vi "Set Default Characteristics.vi"(8 "error in (no error)":errorcluster, 11 "5105 in":refnum<class "5105.lvclass">) -> (0 "error out":errorcluster, 3 "5105 out":refnum<class "5105.lvclass">)   [LabVIEW 2019, in "5105.lvlib" / "5105.lvclass"]
uses:
  5105.lvclass
  C:/Users/rdexter/Documents/Development/PPL/Oscilloscope.lvlibp/Oscilloscope.lvclass
  builds/Instruments/Oscilloscope.lvlibp/Custom Controls/Trigger Modifier.ctl
  builds/Instruments/Oscilloscope.lvlibp/Custom Controls/Trigger Type.ctl
  builds/Instruments/Oscilloscope.lvlibp/Accessors/Read Trigger Settings.vi
  builds/Instruments/Oscilloscope.lvlibp/Accessors/Read Horizontal Setting.vi
  builds/Instruments/Oscilloscope.lvlibp/Accessors/Read Channel Setting.vi
  builds/Instruments/Oscilloscope.lvlibp/Accessors/Write Trigger Settings.vi
  builds/Instruments/Oscilloscope.lvlibp/Accessors/Write Horizontal Setting.vi
  builds/Instruments/Oscilloscope.lvlibp/Accessors/Write Channel Settings.vi
  builds/Instruments/Oscilloscope.lvlibp/Oscilloscope.lvclass
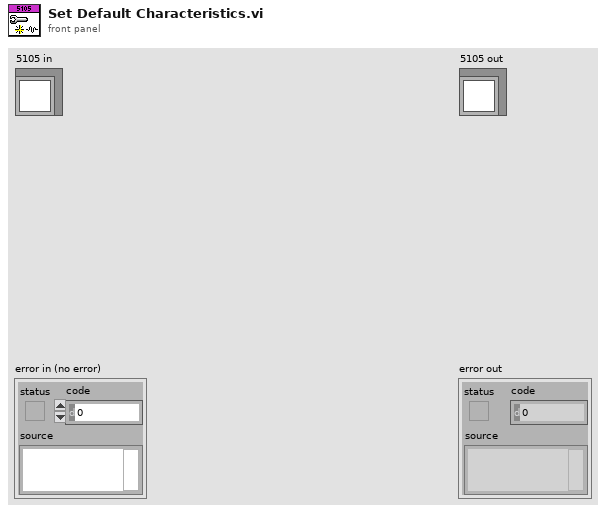
[diagram p1: front panel]
types:
  T1 = typedef "Oscilloscope.lvlibp/Oscilloscope.lvclass/Trigger Type.ctl" = enum16{"Immediate", "Analog Edge", "Digital", "Window", "Hysteresis"}
  T2 = typedef "Oscilloscope.lvlibp/Oscilloscope.lvclass/Trigger Modifier.ctl" = enum16{"Invalid_Setting", "None", "Auto Trigger"}
  T3 = typedef "Oscilloscope.lvlibp/Oscilloscope.lvclass/Trigger Settings.ctl" = cluster{"Edge:":T4, "Level":dbl, "Source":T5, "trigger coupling":T6, "Holdoff":dbl, "Delay":dbl, "Trigger Modifier":T2, "Trigger Type":T1}
  T4 = typedef "Oscilloscope.lvlibp/Oscilloscope.lvclass/Edge Select.ctl" = u16
  T5 = typedef "Oscilloscope.lvlibp/Oscilloscope.lvclass/Channel List.ctl" = u16
  T6 = typedef "Oscilloscope.lvlibp/Oscilloscope.lvclass/Trigger Coupling.ctl" = u16
  T7 = typedef "Oscilloscope.lvlibp/Oscilloscope.lvclass/Horizontal Setting.ctl" = cluster{"Num Records":i32, "Sample Rate":dbl, "Reference Pos":dbl, "Min Record len":i32}
  T8 = typedef "Oscilloscope.lvlibp/Oscilloscope.lvclass/Channel Settings.ctl" = cluster{"Amplitude":dbl, "Vertical Coupling":T9, "Probe Attenuation":dbl, "Enable?":bool, "Maximum Input Frequency":dbl, "Input Impedance":u16, "Timeout (s)":dbl}
  T9 = typedef "Oscilloscope.lvlibp/Oscilloscope.lvclass/Vertical Coupling.ctl" = enum16{"AC", "DC", "Ground"}
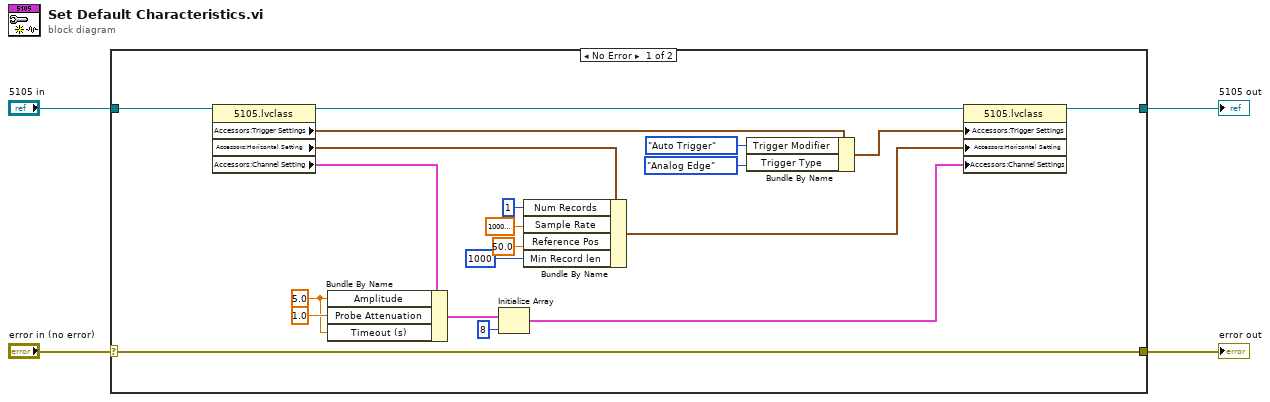
[diagram p0: block diagram]
diagram:
  n1 = case shown="No Error" "error in (no error)" {
    selector: "error in (no error)" -> [w23 w26]
    tunnel: [w23 w26] -> w3
    tunnel: [w24 w25] -> w1
    tunnel: "5105 in" -> [w21 w25]
    frame No Error {
      w18 = 5.0 ("Amplitude")
      n2 = property class="5105.lvclass"(reference=w21) -> (reference out=w16:refnum<class "5105.lvclass">, "Accessors:Trigger Settings"=w8:T3, "Accessors:Horizontal Setting"=w11:T7, "Accessors:Channel Setting"=w20:T8)  [unwired: 1 in, 1 out]
      n3 = Bundle By Name(cluster=w20, "Amplitude"=w18, "Probe Attenuation"=1.0, "Timeout (s)"=w18) -> (w17:T8)
      n4 = Initialize Array(w17, 8 ("dimension size")) -> (w5:T8[])
      n5 = Bundle By Name(cluster=w11, "Num Records"=1, "Sample Rate"=10000000.0, "Reference Pos"=50.0, "Min Record len"=1000) -> (w6:T7)
      n6 = Bundle By Name(cluster=w8, "Trigger Modifier"=Trigger_Modifier."Auto Trigger", "Trigger Type"=Trigger_Type."Analog Edge") -> (w7:T3)
      n7 = property class="5105.lvclass"(reference=w16, "Accessors:Trigger Settings"=w7, "Accessors:Horizontal Setting"=w6, "Accessors:Channel Settings"=w5) -> (reference out=w24:refnum<class "5105.lvclass">)  [unwired: 1 in, 1 out]
    }
    frame Error {
    }
  }
  "error out" <- w3
  "5105 out" <- w1
